vi "Menu.vi"() -> ()   [LabVIEW 2025]
uses:
  <vilib>/Utility/miscctls.llb/LVComboBoxStrsAndValuesArrayTypeDef.ctl
  Controls/Global.vi
panel:
  out "net address":u32
  in  "PageEnum":enum16{"Default", "ServerLobby", "JoinLobby"}(ring)
  in  "isJoinGameLocal":bool
  in  "isHostLocal":bool
  in  "JoinServer Button":bool
  in  "CreateServer Button":bool
  in  "Enter IP":string
  in  "Select Network":string(combo)
  in  "StartGame Button":bool
  out "StartGameText":picture
  out "TitleText":picture
  out "LobbyPlayerCountNumText":picture
  out "PlayerCountText":picture
  out "WaitingText":picture
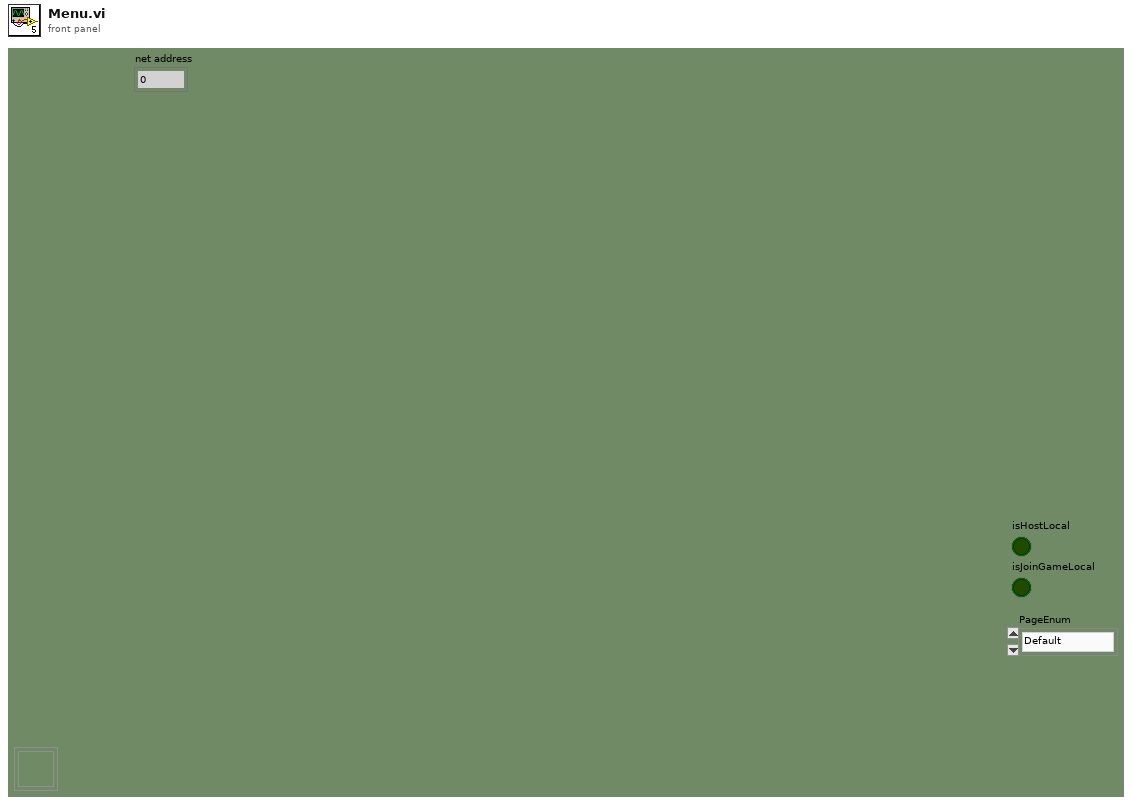
[diagram p1: front panel]
types:
  T1 = enum8{"Enabled", "Disabled", "Disabled and Grayed Out"}
  T2 = typedef "LVComboBoxStrsAndValuesArrayTypeDef.ctl" = cluster{"String":string, "Value":string}[]
  T3 = typedef "imagedata.ctl" = cluster{"image type":i32, "image depth":i32, "image":u8[], "mask":u8[], "colors":u32[], "Rectangle":cluster{"left":i16, "top":i16, "right":i16, "bottom":i16}}
  T4 = typedef "LVBoundsTypeDef.ctl" = cluster{"Width":u32, "Height":u32}
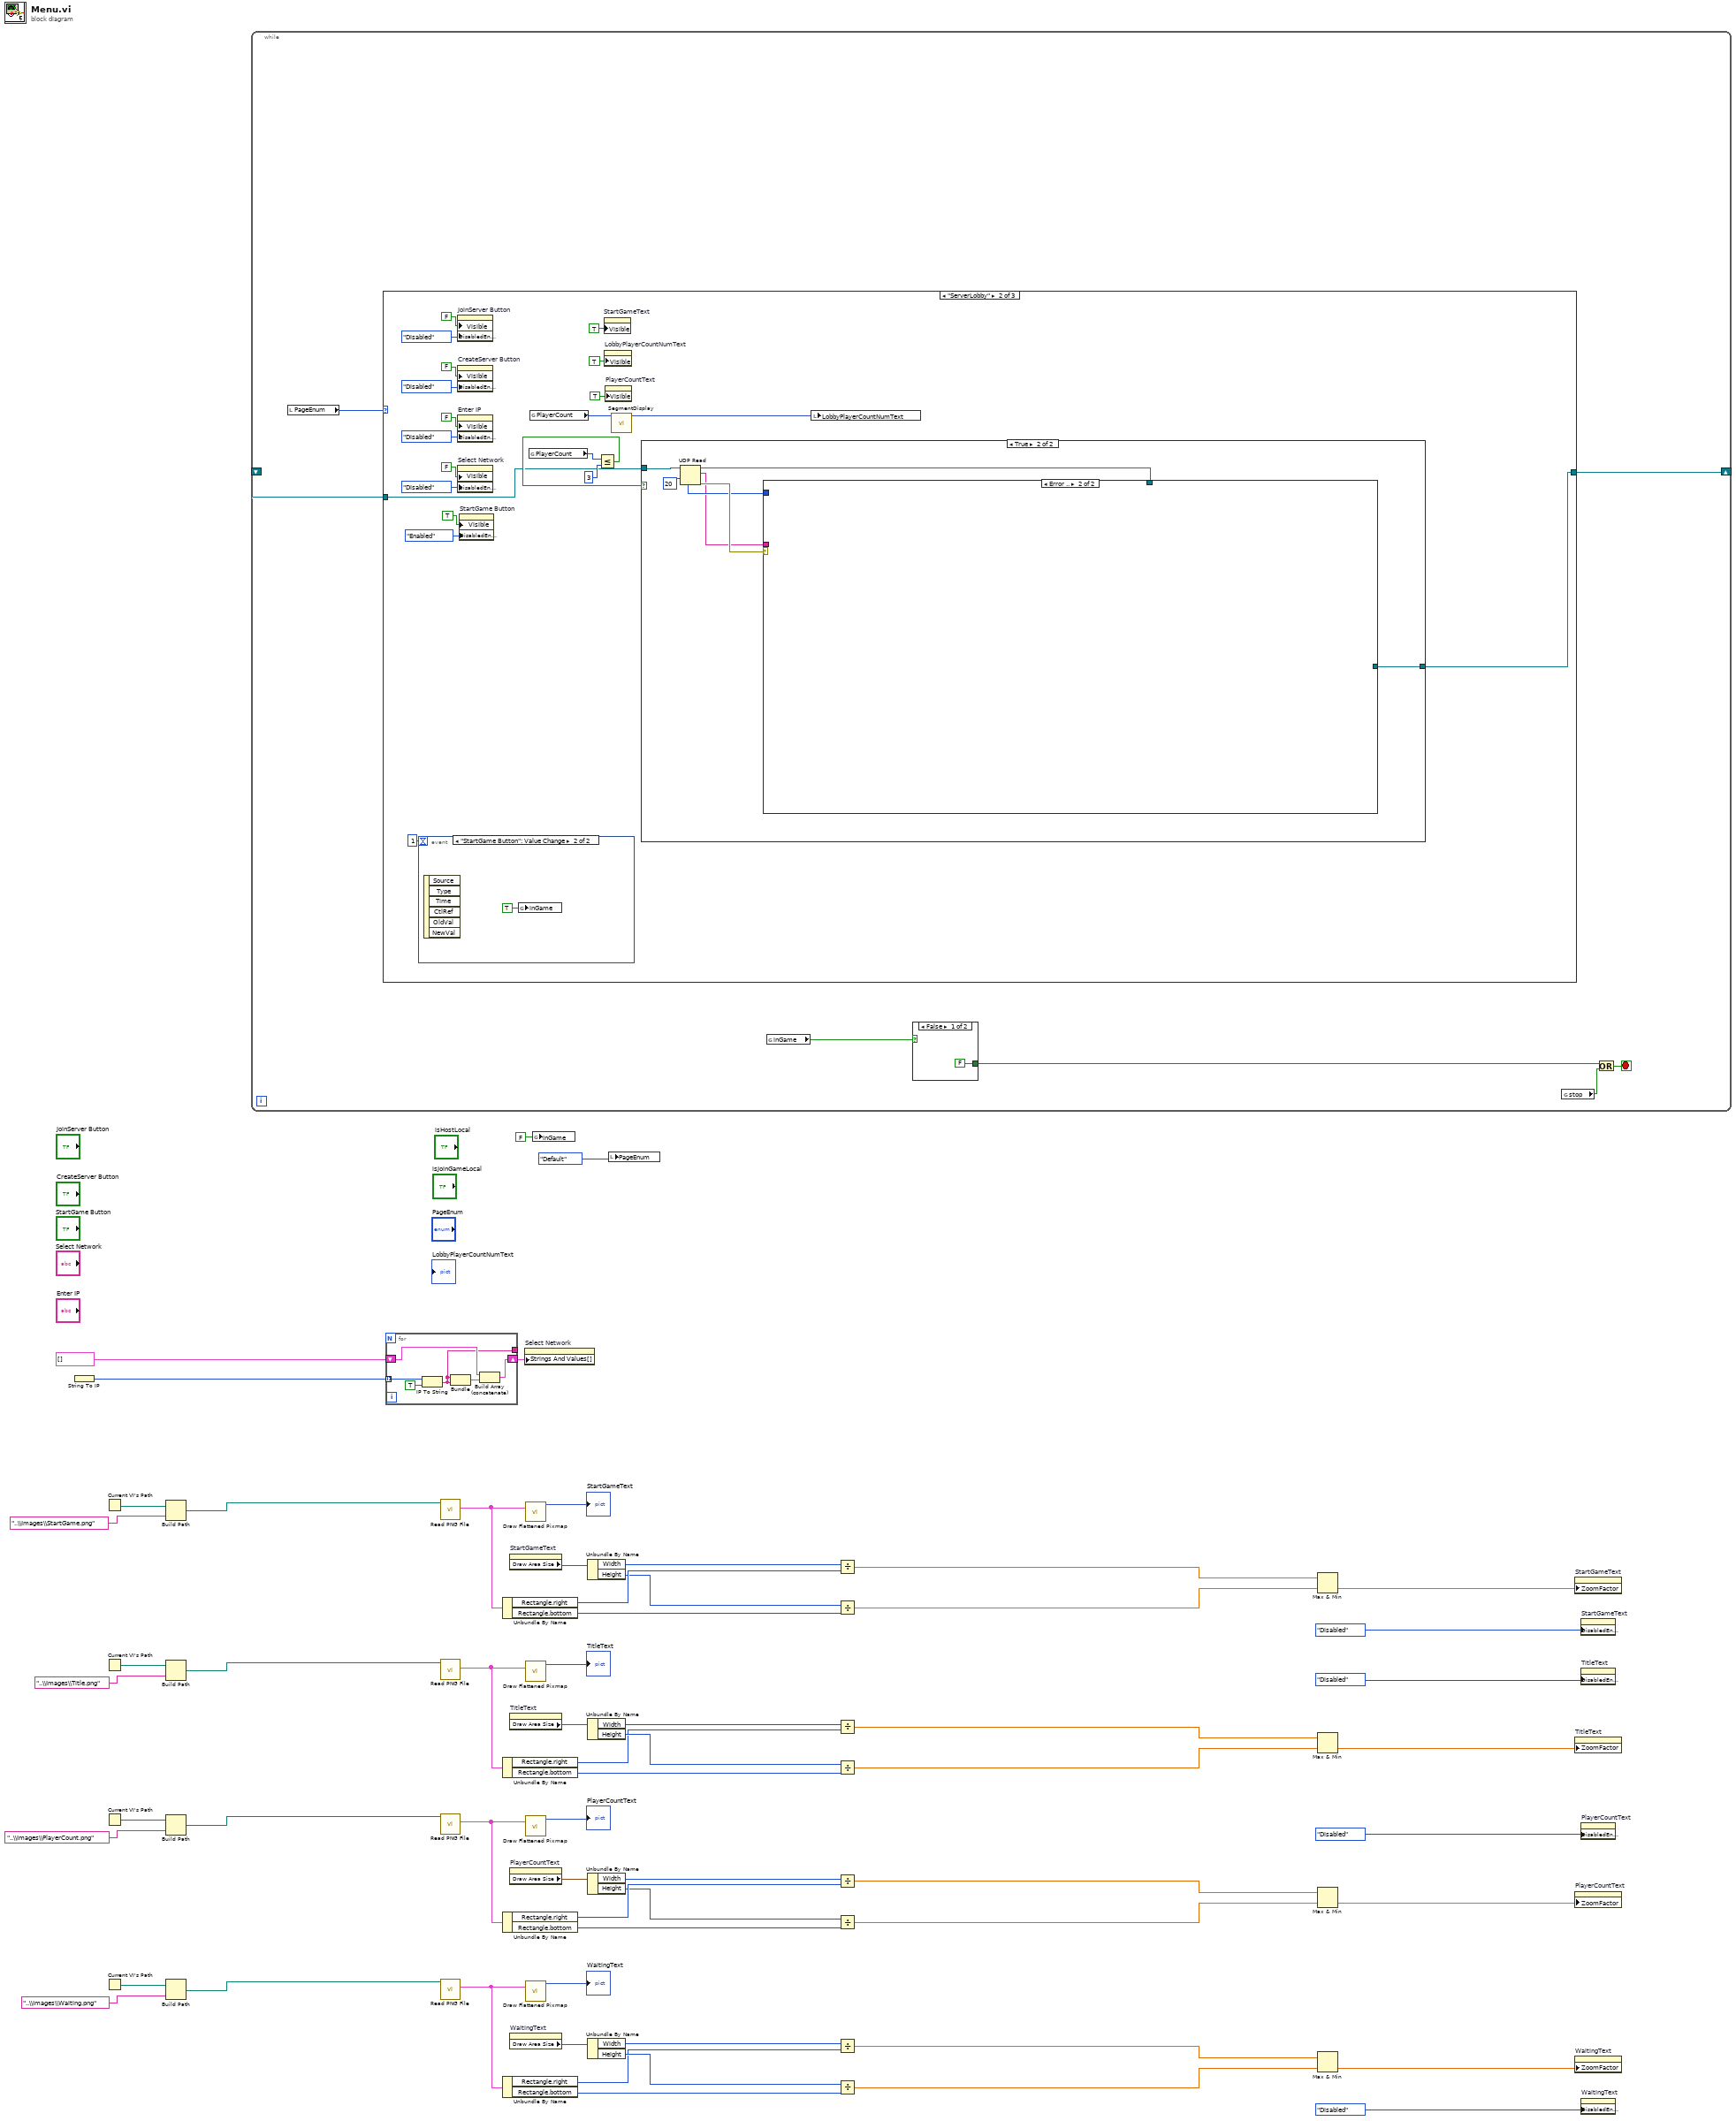
[diagram p0: block diagram]
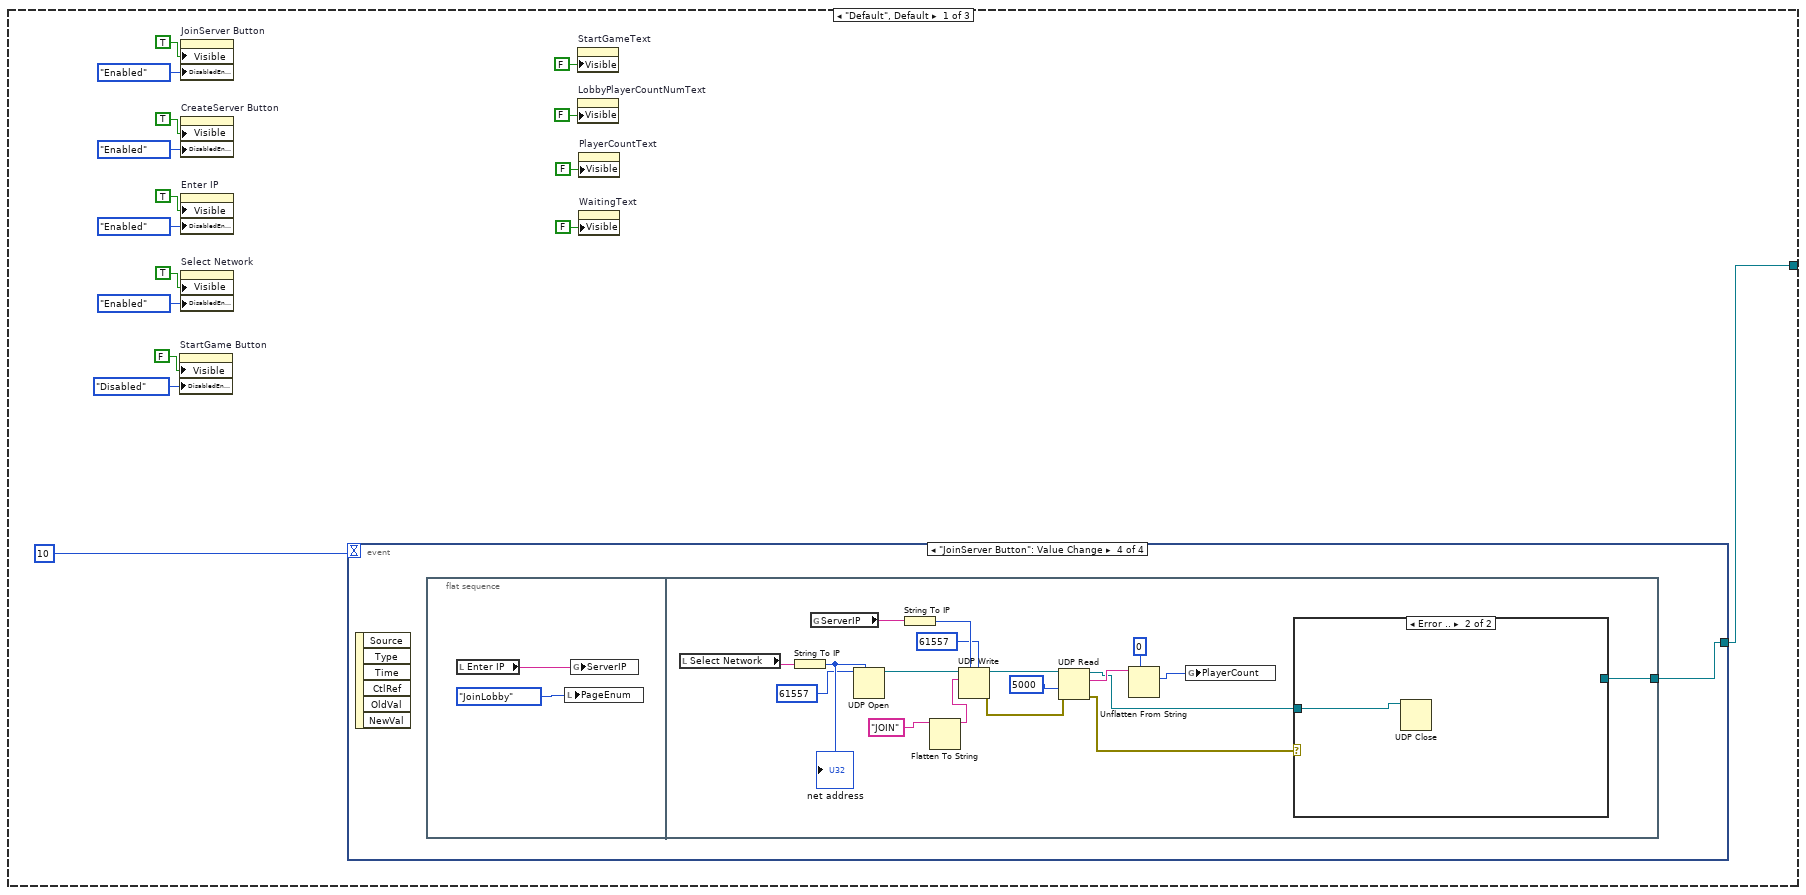
[diagram p2: hidden frame]
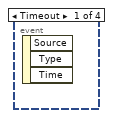
[diagram p3: hidden frame]
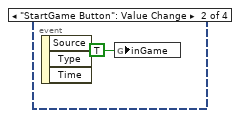
[diagram p4: hidden frame]
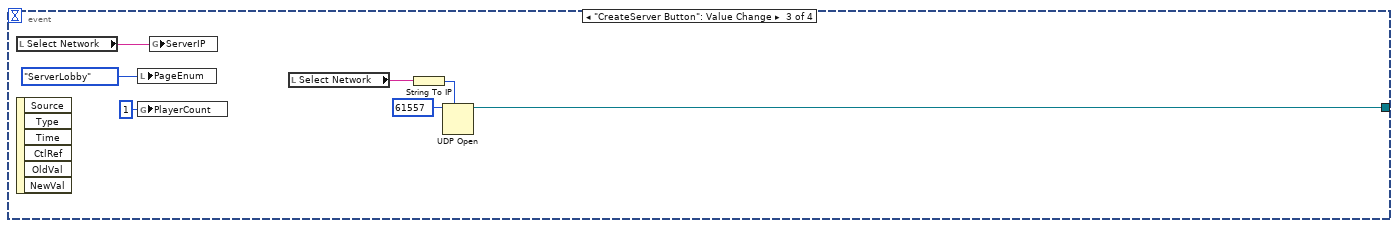
[diagram p5: hidden frame]
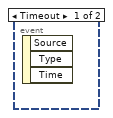
[diagram p7: hidden frame]
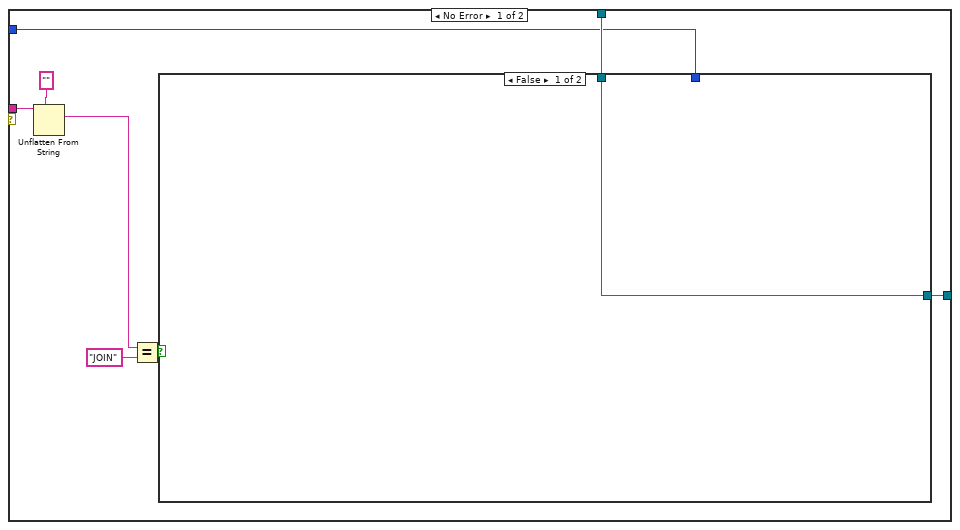
[diagram p9: hidden frame]
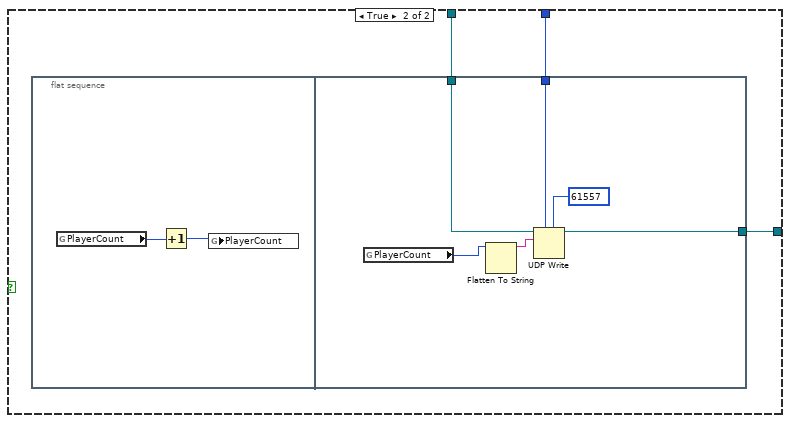
[diagram p10: hidden frame]
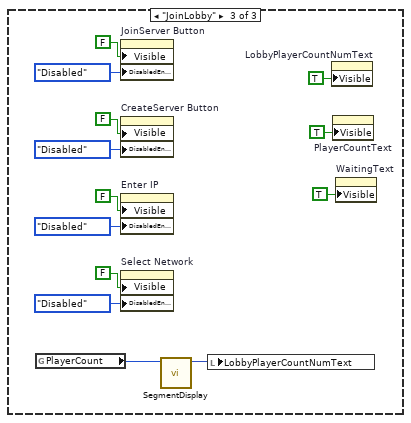
[diagram p11: hidden frame]
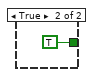
[diagram p12: hidden frame]
diagram:
  n1 = String To IP() -> (0:w61:u32[])  [unwired: 1 in]
  n2 = Current VI's Path() -> (path=w54:path)
  n3 = Current VI's Path() -> (path=w33:path)
  n4 = Current VI's Path() -> (path=w25:path)
  n5 = Current VI's Path() -> (path=w3:path)
  n6 = Build Path(base path=w54, name or relative path="..\\Images\\StartGame.png") -> (appended path=w56:path)
  n7 = Build Path(base path=w33, name or relative path="..\\Images\\Title.png") -> (appended path=w31:path)
  n8 = Build Path(base path=w25, name or relative path="..\\Images\\PlayerCount.png") -> (appended path=w27:path)
  n9 = Build Path(base path=w3, name or relative path="..\\Images\\Waiting.png") -> (appended path=w1:path)
  n10 = while {
    shift-right: [w62] -> _
    shift-left: _ -> [w63]
    stop <- w68 stop-if-true
    n11 = local read "PageEnum"() -> (w64:enum16{"Default", "ServerLobby", "JoinLobby"})
    n12 = case shown="\"ServerLobby\"" w64 {
      tunnel: w63 -> [_ w118 _]
      tunnel: [w69 w116 _] -> w62
      frame "Default", Default {
        n13 = property on="StartGame Button" class="Bool"("Visible"=FALSE, "DisabledEnum"=T1."Disabled" ("Disabled")) -> ()  [unwired: 2 in, 2 out]
        n14 = property on="JoinServer Button" class="Bool"("Visible"=TRUE, "DisabledEnum"=T1."Enabled" ("Disabled")) -> ()  [unwired: 2 in, 2 out]
        n15 = property on="CreateServer Button" class="Bool"("Visible"=TRUE, "DisabledEnum"=T1."Enabled" ("Disabled")) -> ()  [unwired: 2 in, 2 out]
        n16 = property on="Enter IP" class="Str"("Visible"=TRUE, "DisabledEnum"=T1."Enabled" ("Disabled")) -> ()  [unwired: 2 in, 2 out]
        n17 = property on="Select Network" class="CmbBox"("Visible"=TRUE, "DisabledEnum"=T1."Enabled" ("Disabled")) -> ()  [unwired: 2 in, 2 out]
        n18 = event shown="[3] \"JoinServer Button\": Value Change" {
          selector: _ -> [_ _ _ _]
          dyn-events: _ -> [_ _ _ _]
          timeout: 10 -> [_ _ _ _]
          tunnel: [_ _ w86 w93] -> w69
          event Timeout {
            n19 = event-data() -> ()  [unwired: 1 in, 3 out]
          }
          event "StartGame Button": Value Change {
            n20 = event-data() -> ()  [unwired: 1 in, 3 out]
            n21 = global write "Global.vi" "inGame"(TRUE) -> ()
          }
          event "CreateServer Button": Value Change {
            n22 = local read "Select Network"() -> (w92:string)
            n23 = event-data() -> ()  [unwired: 1 in, 6 out]
            n24 = local write "PageEnum"(enum16{"Default", "ServerLobby"}."ServerLobby") -> ()
            n25 = global write "Global.vi" "PlayerCount"(u32 1 ("PlayerCount")) -> ()
            n26 = global write "Global.vi" "ServerIP"(w92) -> ()
            n27 = local read "Select Network"() -> (w89:string)
            n28 = String To IP(1:w89) -> (0:w87:u32)
            n29 = UDP Open(7:w87, 11:u16 61557 ("port")) -> (port=w86:refnum<k16>)  [unwired: 3 in, 2 out]
          }
          event "JoinServer Button": Value Change {
            n30 = event-data() -> ()  [unwired: 1 in, 6 out]
            n31 = flat-sequence {
              tunnel: [w96] -> w93
              frame #0 {
                n32 = local read "Enter IP"() -> (w95:string)
                n33 = local write "PageEnum"(enum16{"Default", "ServerLobby", "JoinLobby"}."JoinLobby" ("PageEnum")) -> ()
                n34 = global write "Global.vi" "ServerIP"(w95) -> ()
              }
              frame #1 {
                n35 = local read "Select Network"() -> (w113:string)
                n36 = String To IP(1:w113) -> (0:w112:u32)
                "net address" <- w112
                n37 = global read "Global.vi" "ServerIP"() -> (w110:string)
                n38 = UDP Open(7:w112, 11:u16 61557 ("port")) -> (port=w108:refnum<k16>)  [unwired: 3 in, 2 out]
                n39 = String To IP(1:w110) -> (0:w109:u32)
                n40 = Flatten To String(anything="JOIN" ("data in")) -> (data string=w98:string)  [unwired: 3 in, 2 out]
                n41 = UDP Write(address=w109, port or service name=u16 61557, connection ID=w108, data in=w98) -> (error out=w105:errorcluster, 3:w106:refnum<k16>)  [unwired: 2 in]
                n42 = UDP Read(connection ID=w106, timeout ms (25000)=5000, 8:w105) -> (data out=w100:string, error out=w104:errorcluster, 3:w97:refnum<k16>)  [unwired: 1 in, 2 out]
                n43 = Unflatten From String(type=u32 0, binary string=w100) -> (value=w101:u32)  [unwired: 3 in, 2 out]
                n44 = global write "Global.vi" "PlayerCount"(w101) -> ()
                n45 = case shown="Error .." w104 {
                  tunnel: [w114 _] -> w96
                  tunnel: w97 -> [w114 w115]
                  frame No Error {
                  }
                  frame Error {
                    n46 = UDP Close(connection ID=w115) -> ()  [unwired: 1 in, 2 out]
                  }
                }
              }
            }
          }
        }
        n47 = property on="StartGameText" class="Pict"("Visible"=FALSE) -> ()  [unwired: 2 in, 2 out]
        n48 = property on="LobbyPlayerCountNumText" class="Pict"("Visible"=FALSE) -> ()  [unwired: 2 in, 2 out]
        n49 = property on="PlayerCountText" class="Pict"("Visible"=FALSE) -> ()  [unwired: 2 in, 2 out]
        n50 = property on="WaitingText" class="Pict"("Visible"=FALSE) -> ()  [unwired: 2 in, 2 out]
      }
      frame "ServerLobby" {
        n51 = event shown="[1] \"StartGame Button\": Value Change" {
          selector: _ -> [_ _]
          dyn-events: _ -> [_ _]
          timeout: 1 -> [_ _]
          event Timeout {
            n52 = event-data() -> ()  [unwired: 1 in, 3 out]
          }
          event "StartGame Button": Value Change {
            n53 = event-data() -> ()  [unwired: 1 in, 6 out]
            n54 = global write "Global.vi" "inGame"(TRUE) -> ()
          }
        }
        n55 = property on="JoinServer Button" class="Bool"("Visible"=FALSE, "DisabledEnum"=T1."Disabled" ("Disabled")) -> ()  [unwired: 2 in, 2 out]
        n56 = property on="CreateServer Button" class="Bool"("Visible"=FALSE, "DisabledEnum"=T1."Disabled" ("Disabled")) -> ()  [unwired: 2 in, 2 out]
        n57 = property on="Enter IP" class="Str"("Visible"=FALSE, "DisabledEnum"=T1."Disabled" ("Disabled")) -> ()  [unwired: 2 in, 2 out]
        n58 = property on="Select Network" class="CmbBox"("Visible"=FALSE, "DisabledEnum"=T1."Disabled" ("Disabled")) -> ()  [unwired: 2 in, 2 out]
        n59 = property on="StartGame Button" class="Bool"("Visible"=TRUE, "DisabledEnum"=T1."Enabled" ("Disabled")) -> ()  [unwired: 2 in, 2 out]
        n60 = global read "Global.vi" "PlayerCount"() -> (w121:u32)
        n61 = global read "Global.vi" "PlayerCount"() -> (w125:u32)
        n62 = Less Or Equal?(x=w121, y=u32 3) -> (x <= y?=w119:bool)
        n63 = property on="StartGameText" class="Pict"("Visible"=TRUE) -> ()  [unwired: 2 in, 2 out]
        n64 = property on="LobbyPlayerCountNumText" class="Pict"("Visible"=TRUE) -> ()  [unwired: 2 in, 2 out]
        n65 = property on="PlayerCountText" class="Pict"("Visible"=TRUE) -> ()  [unwired: 2 in, 2 out]
        n66 = call "SegmentDisplay.vi"("Numeric"=w125) -> ("new picture"=w122:picture)  [unwired: 10 in]
        n67 = case shown="True" w119 {
          tunnel: w118 -> [_ w144]
          tunnel: [_ w138] -> w116
          frame False {
          }
          frame True {
            n68 = UDP Read(connection ID=w144, timeout ms (25000)=20) -> (data out=w139:string, error out=w142:errorcluster, 3:w141:refnum<k16>, 6:w140:u32)  [unwired: 2 in, 1 out]
            n69 = case shown="Error .." w142 {
              tunnel: w141 -> [w150 _]
              tunnel: w140 -> [w149 _]
              tunnel: w139 -> [w148 _]
              tunnel: [w145 _] -> w138
              frame No Error {
                n70 = Unflatten From String(type="", binary string=w148) -> (value=w147:string)  [unwired: 3 in, 2 out]
                n71 = Equal?(x=w147, y="JOIN") -> (x = y?=w152:bool)
                n72 = case shown="False" w152 {
                  tunnel: w150 -> [w153 w156]
                  tunnel: w149 -> [_ w155]
                  tunnel: [w153 w154] -> w145
                  frame False {
                  }
                  frame True {
                    n73 = flat-sequence {
                      tunnel: w156 -> [w164]
                      tunnel: w155 -> [w161]
                      tunnel: [w159] -> w154
                      frame #0 {
                        n74 = global read "Global.vi" "PlayerCount"() -> (w158:u32)
                        n75 = Increment(x=w158) -> (x+1=w157:u32)
                        n76 = global write "Global.vi" "PlayerCount"(w157) -> ()
                      }
                      frame #1 {
                        n77 = global read "Global.vi" "PlayerCount"() -> (w163:u32)
                        n78 = Flatten To String(anything=w163) -> (data string=w162:string)  [unwired: 3 in, 2 out]
                        n79 = UDP Write(address=w161, port or service name=u16 61557, connection ID=w164, data in=w162) -> (3:w159:refnum<k16>)  [unwired: 2 in, 1 out]
                      }
                    }
                  }
                }
              }
              frame Error {
              }
            }
          }
        }
        n80 = local write "LobbyPlayerCountNumText"(w122) -> ()
      }
      frame "JoinLobby" {
        n81 = global read "Global.vi" "PlayerCount"() -> (w169:u32)
        n82 = property on="JoinServer Button" class="Bool"("Visible"=FALSE, "DisabledEnum"=T1."Disabled" ("Disabled")) -> ()  [unwired: 2 in, 2 out]
        n83 = property on="CreateServer Button" class="Bool"("Visible"=FALSE, "DisabledEnum"=T1."Disabled" ("Disabled")) -> ()  [unwired: 2 in, 2 out]
        n84 = property on="Enter IP" class="Str"("Visible"=FALSE, "DisabledEnum"=T1."Disabled" ("Disabled")) -> ()  [unwired: 2 in, 2 out]
        n85 = property on="Select Network" class="CmbBox"("Visible"=FALSE, "DisabledEnum"=T1."Disabled" ("Disabled")) -> ()  [unwired: 2 in, 2 out]
        n86 = call "SegmentDisplay.vi"("Numeric"=w169) -> ("new picture"=w168:picture)  [unwired: 10 in]
        n87 = local write "LobbyPlayerCountNumText"(w168) -> ()
        n88 = property on="LobbyPlayerCountNumText" class="Pict"("Visible"=TRUE) -> ()  [unwired: 2 in, 2 out]
        n89 = property on="PlayerCountText" class="Pict"("Visible"=TRUE) -> ()  [unwired: 2 in, 2 out]
        n90 = property on="WaitingText" class="Pict"("Visible"=TRUE) -> ()  [unwired: 2 in, 2 out]
      }
    }
    n91 = global read "Global.vi" "inGame"() -> (w65:bool)
    n92 = case shown="False" w65 {
      tunnel: [FALSE TRUE] -> w67
      frame False {
      }
      frame True {
      }
    }
    n93 = global read "Global.vi" "stop"() -> (w66:bool)
    n94 = Or(x=w67, y=w66) -> (x .or. y?=w68:bool)
  }
  n95 = for {
    tunnel: w61 -> [w182] mode=indexing
    shift-right: [w184] -> w59
    shift-left: T2 [] ("Strings And Values []") -> [w185]
    tunnel: [w180] -> _
    n96 = IP To String(1:TRUE ("dot notation? (F)"), 2:w182) -> (0:w180:string)
    n97 = Bundle("name"=w180, "name"=w180) -> (w181:cluster{"name":string, "name":string})  [unwired: 1 in]
    n98 = Build Array (concatenate)(w185, w181) -> (w184:T2)
  }
  n99 = call <vilib>:"Read PNG File.vi"("path to PNG file"=w56) -> ("image data"=w45:T3)  [unwired: 8 in, 2 out]
  n100 = call <vilib>:"Read PNG File.vi"("path to PNG file"=w31) -> ("image data"=w42:T3)  [unwired: 8 in, 2 out]
  n101 = call <vilib>:"Read PNG File.vi"("path to PNG file"=w27) -> ("image data"=w16:T3)  [unwired: 8 in, 2 out]
  n102 = call <vilib>:"Read PNG File.vi"("path to PNG file"=w1) -> ("image data"=w12:T3)  [unwired: 8 in, 2 out]
  n103 = Unbundle By Name(w45) -> ("Rectangle.right"=w50:i16, "Rectangle.bottom"=w53:i16)
  n104 = Unbundle By Name(w42) -> ("Rectangle.right"=w37:i16, "Rectangle.bottom"=w34:i16)
  n105 = Unbundle By Name(w16) -> ("Rectangle.right"=w21:i16, "Rectangle.bottom"=w24:i16)
  n106 = Unbundle By Name(w12) -> ("Rectangle.right"=w7:i16, "Rectangle.bottom"=w4:i16)
  n107 = property on="StartGameText" class="Pict"() -> ("Draw Area Size"=w52:T4)  [unwired: 2 in, 2 out]
  n108 = property on="TitleText" class="Pict"() -> ("Draw Area Size"=w35:T4)  [unwired: 2 in, 2 out]
  n109 = property on="PlayerCountText" class="Pict"() -> ("Draw Area Size"=w23:T4)  [unwired: 2 in, 2 out]
  n110 = property on="WaitingText" class="Pict"() -> ("Draw Area Size"=w5:T4)  [unwired: 2 in, 2 out]
  n111 = property on="Select Network" class="CmbBox"("Strings And Values[]"=w59) -> ()  [unwired: 2 in, 2 out]
  n112 = call <vilib>:"Draw Flattened Pixmap.vi"("image data"=w45) -> ("new picture"=→"StartGameText":picture)  [unwired: 8 in]
  n113 = call <vilib>:"Draw Flattened Pixmap.vi"("image data"=w42) -> ("new picture"=→"TitleText":picture)  [unwired: 8 in]
  n114 = call <vilib>:"Draw Flattened Pixmap.vi"("image data"=w16) -> ("new picture"=→"PlayerCountText":picture)  [unwired: 8 in]
  n115 = call <vilib>:"Draw Flattened Pixmap.vi"("image data"=w12) -> ("new picture"=→"WaitingText":picture)  [unwired: 8 in]
  n116 = global write "Global.vi" "inGame"(FALSE) -> ()
  n117 = Unbundle By Name(w52) -> ("Width"=w51:u32, "Height"=w49:u32)
  n118 = Unbundle By Name(w35) -> ("Width"=w36:u32, "Height"=w38:u32)
  n119 = Unbundle By Name(w23) -> ("Width"=w22:u32, "Height"=w20:u32)
  n120 = Unbundle By Name(w5) -> ("Width"=w6:u32, "Height"=w8:u32)
  n121 = local write "PageEnum"(enum16{"Default", "ServerLobby", "JoinLobby"}."Default") -> ()
  n122 = Divide(x=w51, y=w50) -> (x/y=w48:dbl)
  n123 = Divide(x=w49, y=w53) -> (x/y=w47:dbl)
  n124 = Divide(x=w36, y=w37) -> (x/y=w39:dbl)
  n125 = Divide(x=w38, y=w34) -> (x/y=w40:dbl)
  n126 = Divide(x=w22, y=w21) -> (x/y=w19:dbl)
  n127 = Divide(x=w20, y=w24) -> (x/y=w18:dbl)
  n128 = Divide(x=w6, y=w7) -> (x/y=w9:dbl)
  n129 = Divide(x=w8, y=w4) -> (x/y=w10:dbl)
  n130 = Max & Min(x=w48, y=w47) -> (min(x,y)=w46:dbl)  [unwired: 1 out]
  n131 = Max & Min(x=w39, y=w40) -> (min(x,y)=w41:dbl)  [unwired: 1 out]
  n132 = Max & Min(x=w19, y=w18) -> (min(x,y)=w17:dbl)  [unwired: 1 out]
  n133 = Max & Min(x=w9, y=w10) -> (min(x,y)=w11:dbl)  [unwired: 1 out]
  n134 = property on="StartGameText" class="Pict"("ZoomFactor"=w46) -> ()  [unwired: 2 in, 2 out]
  n135 = property on="TitleText" class="Pict"("ZoomFactor"=w41) -> ()  [unwired: 2 in, 2 out]
  n136 = property on="PlayerCountText" class="Pict"("ZoomFactor"=w17) -> ()  [unwired: 2 in, 2 out]
  n137 = property on="WaitingText" class="Pict"("ZoomFactor"=w11) -> ()  [unwired: 2 in, 2 out]
  n138 = property on="StartGameText" class="Pict"("DisabledEnum"=T1."Disabled" ("Disabled")) -> ()  [unwired: 2 in, 2 out]
  n139 = property on="TitleText" class="Pict"("DisabledEnum"=T1."Disabled" ("Disabled")) -> ()  [unwired: 2 in, 2 out]
  n140 = property on="PlayerCountText" class="Pict"("DisabledEnum"=T1."Disabled" ("Disabled")) -> ()  [unwired: 2 in, 2 out]
  n141 = property on="WaitingText" class="Pict"("DisabledEnum"=T1."Disabled" ("Disabled")) -> ()  [unwired: 2 in, 2 out]
